vi "ExpScreen (SubVI).vi"(0 "Color Box":u32(colorbox)=16763225, 1 "go in":bool, 2 "end in":bool, 3 "value in":dbl, 4 "%MVC in":dbl) -> ()   [LabVIEW 2011]
panel:
  out "GO":bool
  out "END":bool
  out "Target":dbl(slide)=25.0 scale=0.0..60.0
  out "%MVC out":dbl(slide)=inf scale=0.0..60.0
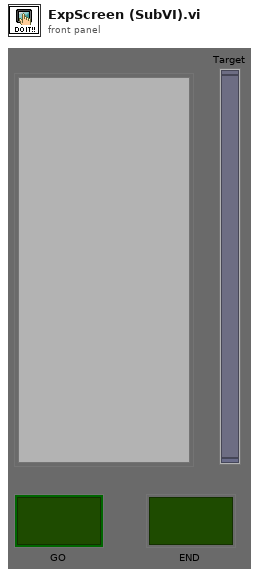
[diagram p1: front panel]
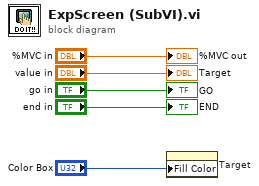
[diagram p0: block diagram]
diagram:
  n1 = property on="Target" class="Slide (strict)"("Fill Color"="Color Box") -> ()  [unwired: 2 in, 2 out]
  "%MVC out" <- "%MVC in"
  "Target" <- "value in"
  "END" <- "end in"
  "GO" <- "go in"
